vi "Sea-Level SWI Set Stimulus.vi"(7 "Sea-Level SWI":T2, 8 "error in (no error)":errorcluster, 10 "SWI Position":T1, 11 "Handle":i32) -> (0 "error out":errorcluster, 3 "Handle Out":i32)   [LabVIEW 2011]
uses:
  TypeDefs/Sea-Level SWI Adapter Info.ctl
  TypeDefs/Sea-Level SWI Position.ctl
  TypeDefs/Sea-Level SWI Access Mode.ctl
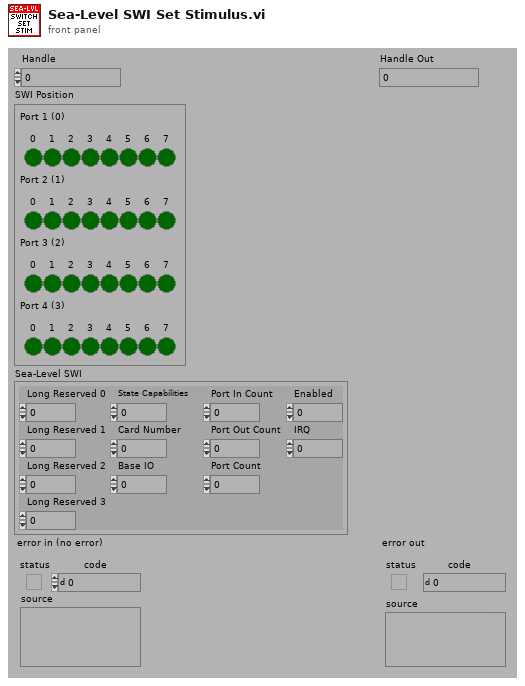
[diagram p1: front panel]
types:
  T1 = typedef "Sea-Level SWI Position.ctl" = cluster{"Port 1 (0)":cluster{"0":bool, "1":bool, "2":bool, "3":bool, "4":bool, "5":bool, "6":bool, "7":bool}, "Port 2 (1)":cluster{"0":bool, "1":bool, "2":bool, "3":bool, "4":bool, "5":bool, "6":bool, "7":bool}, "Port 3 (2)":cluster{"0":bool, "1":bool, "2":bool, "3":bool, "4":bool, "5":bool, "6":bool, "7":bool}, "Port 4 (3)":cluster{"0":bool, "1":bool, "2":bool, "3":bool, "4":bool, "5":bool, "6":bool, "7":bool}}
  T2 = typedef "Sea-Level SWI Adapter Info.ctl" = cluster{"Long Reserved 0":i32, "Long Reserved 1":i32, "Long Reserved 2":i32, "Long Reserved 3":i32, "State Capabilities":i32, "Card Number":i16, "Base IO":i16, "Port In Count":i8, "Port Out Count":i8, "Port Count":i8, "Enabled":i8, "IRQ":i16}
  T3 = typedef "Sea-Level SWI Access Mode.ctl" = enum16{"Relative", "Absolute"}
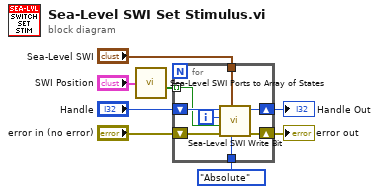
[diagram p0: block diagram]
diagram:
  n1 = call "Sea-Level SWI Ports to Array of States.vi"("SWI Position"="SWI Position") -> ("State Array"=w1:bool[])  [unwired: 7 out]
  n2 = for {
    tunnel: "Sea-Level SWI" -> [w12]
    tunnel: Sea-Level_SWI_Access_Mode."Absolute" ("Access Mode (Relative)") -> [w11]
    shift-right: [w13] -> w3
    shift-left: "Handle" -> [w15]
    shift-right: [w14] -> w4
    shift-left: "error in (no error)" -> [w16]
    tunnel: w1 -> [w10] mode=indexing
    i -> [w9]
    n3 = call "Sea-Level SWI Write Bit.vi"("Access Mode (Relative)"=w11, "Adapter Info"=w12, "error in (no error)"=w16, "State"=w10, "Bit Number"=w9, "Handle"=w15) -> ("error out"=w14:errorcluster, "Handle Out"=w13:i32)  [unwired: 4 out]
  }
  "error out" <- w4
  "Handle Out" <- w3
